vi "3-4.vi"   [LabVIEW 2022 SP3]
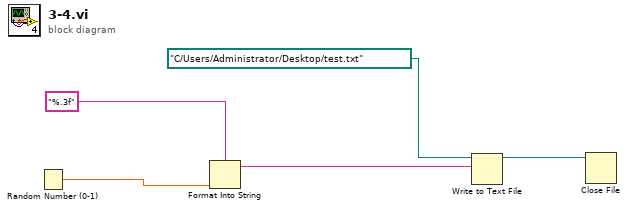
[diagram p0: block diagram]
diagram:
  n1 = Random Number (0-1)() -> (number: 0 to 1=w5:dbl)
  n2 = Format Into String(format string="%.3f", w5) -> (resulting string=w3:string)  [unwired: 2 in, 1 out]
  n3 = Write to Text File(file (use dialog)=path "C:/Users/Administrator/Desktop/test.txt" ("文件（使用对话框）"), text=w3) -> (refnum out=w2:refnum<file>)  [unwired: 2 in, 2 out]
  n4 = Close File(refnum=w2) -> ()  [unwired: 1 in, 2 out]
